vi "Write Registers.vi"(8 "error in (no error)":errorcluster, 11 "Serial Config":T1={"串口选择"="", "通讯速率"=9600, "超时时间"=200, "数据位长"=8, "奇偶校验"=enum."None", "停止位长"=10, "握手控制"=0, "字符结束"=TRUE, "结束字符"=10, "仪器地址"=1} {"结束字符" format="%.0x"; "握手控制" items=["None", "XON/XOFF", "RTS/CTS", "XON/XOFF & RTS/CTS", "DTR/DSR", "XON/XOFF & DTR/DSR"]; "停止位长" items=["1.0"=10, "1.5"=15, "2.0"=20]; "数据位长" min=5 max=8 step=1}) -> (0 "error out":errorcluster, 3 "Status Code":string)   [LabVIEW 2010, in "DCP551.lvlib"]
uses:
  DCP551.lvlib
  <vilib>/Instr/_visa.llb/VISA Configure Serial Port (Instr).vi
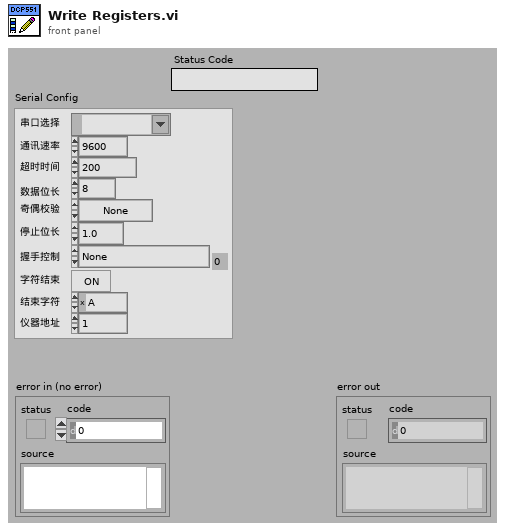
[diagram p1: front panel]
types:
  T1 = cluster{"串口选择":refnum<visa-resource-name>, "通讯速率":u32, "超时时间":u32, "数据位长":u16, "奇偶校验":enum16{"None", "Odd", "Even", "Mark", "Space"}, "停止位长":u16, "握手控制":u16, "字符结束":bool, "结束字符":u8, "仪器地址":u32}
  T2 = cluster{"261W":string, "262W":string, "263W":string, "264W":string, "265W":string}
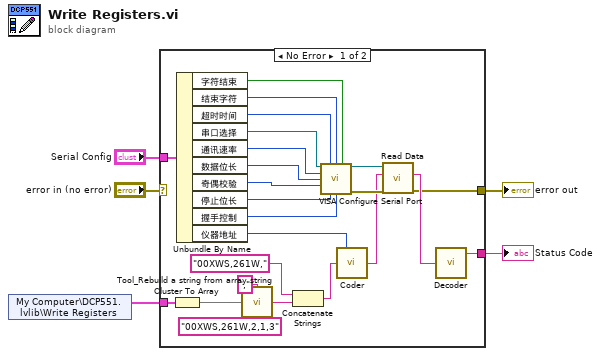
[diagram p0: block diagram]
diagram:
  n1 = shared-variable "My Computer\\DCP551.lvlib\\Write Registers"() -> (w1:T2)  [unwired: 1 in, 1 out]
  n2 = case shown="No Error" "error in (no error)" {
    selector: "error in (no error)" -> [_ w29]
    tunnel: "Serial Config" -> [w19 _]
    tunnel: [w14 w29] -> w3
    tunnel: [w13 _] -> w2
    tunnel: w1 -> [w11 _]
    frame No Error {
      (unwired) "00XWS,261W,2,1,3" ("string")
      n3 = Cluster To Array(cluster=w11) -> (array=w7:string[])
      n4 = Unbundle By Name(w19) -> ("字符结束"=w22:bool, "结束字符"=w21:u8, "超时时间"=w20:u32, "串口选择"=w28:refnum<visa-resource-name>, "通讯速率"=w27:u32, "数据位长"=w26:u16, "奇偶校验"=w25:enum16{"None", "Odd", "Even", "Mark", "Space"}, "停止位长"=w24:u16, "握手控制"=w23:u16, "仪器地址"=w12:u32)
      n5 = call "Tool_Rebuild a string from array string.vi"("Delimiter"=",", "String Array"=w7) -> ("String"=w8:string)  [unwired: 13 in]
      n6 = Concatenate Strings("00XWS,261W," ("string"), w8) -> (w6:string)
      n7 = call-poly "VISA Configure Serial Port"("VISA resource name"=w28, "timeout (10sec)"=w20, "termination char\n(0xA = '\\n' = LF)"=w21, "Enable Termination\nChar (T)"=w22, "baud rate (9600)"=w27, "data bits (8)"=w26, "parity (0:none)"=w25, "stop bits (10: 1 bit)"=w24, "flow control (0:none)"=w23) -> ("VISA resource name out"=w18:refnum<visa-resource-name>, "error out"=w17:errorcluster)  [unwired: 1 in, 4 out]
      n8 = call "Coder.vi"("Station Address"=w12, "Input"=w6) -> ("Output"=w16:string)  [unwired: 13 in]
      n9 = call "Read Data.vi"("error in (no error)"=w17, "COMMAND"=w16, "VISA resource name in"=w18) -> ("error out"=w14:errorcluster, "Output"=w15:string)  [unwired: 6 in, 1 out]
      n10 = call "Decoder.vi"("Input"=w15) -> ("Status Code"=w13:string)  [unwired: 1 out]
    }
    frame Error {
    }
  }
  "error out" <- w3
  "Status Code" <- w2
